vi "ESA-C Move Absolute.vi"(1 "Running":refnum<vi>, 3 "Drive New Abs. Positions":T1={"Drive X Set"=10.0, "Drive Y Set"=10.0, "Drive Z Set"=10.0} {"Drive X Set" min=10.0 max=160.0 step=0.1 format="%.1f"; "Drive Z Set" min=10.0 max=160.0 step=0.1 format="%.1f"; "Drive Y Set" min=10.0 max=160.0 step=0.1 format="%.1f"}, 4 "Drive Connection Settings":T2={"Objective GPIB-Port"=4, "Stage GPIB-Port"=4, "Drive Selector"=0, "Drive Velocity (V/s)"=5.0} {"Drive Velocity (V/s)" min=10.0 max=160.0 step=0.1 format="%.1f"; "Drive Selector" items=["Obj.", "Stage"]; "Stage GPIB-Port" min=1 max=20 step=1 format="%#.0f"; "Objective GPIB-Port" min=1 max=20 step=1 format="%#.0f"}) -> ()   [LabVIEW 2010]
uses:
  TypeDefs/ESA-C Connection Settings.ctl
  TypeDefs/ESA-C Set Positions.ctl
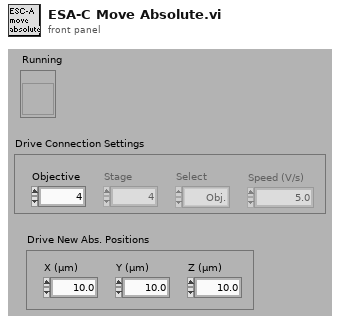
[diagram p1: front panel]
types:
  T1 = typedef "ESA-C Set Positions.ctl" = cluster{"Drive X Set":dbl, "Drive Y Set":dbl, "Drive Z Set":dbl}
  T2 = typedef "ESA-C Connection Settings.ctl" = cluster{"Objective GPIB-Port":i32, "Stage GPIB-Port":i32, "Drive Selector":u16, "Drive Velocity (V/s)":dbl}
  T3 = typedef "ESA-C Current Values.ctl" = cluster{"Voltages":cluster{"Drive X Voltage":dbl, "Drive Y Voltage":dbl, "Drive Z Voltage":dbl}, "Position":cluster{"Drive X Position":dbl, "Drive Y Position":dbl, "Drive Z Position":dbl}}
  T4 = cluster{"Drive X Voltage":dbl, "Drive Y Voltage":dbl, "Drive Z Voltage":dbl}
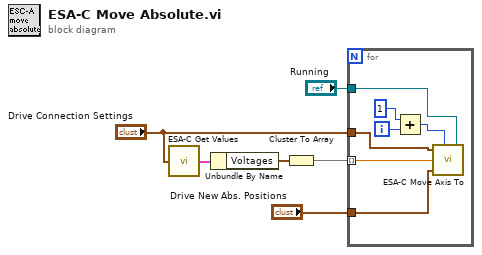
[diagram p0: block diagram]
diagram:
  n1 = call "ESA-C Get Values.vi"("Drive Connection Settings"="Drive Connection Settings") -> ("Drive Current Values"=w6:T3)
  n2 = Unbundle By Name(w6) -> ("Voltages"=w5:T4)
  n3 = Cluster To Array(cluster=w5) -> (array=w4:dbl[])
  n4 = for {
    tunnel: w4 -> [w10] mode=indexing
    tunnel: "Drive New Abs. Positions" -> [w9]
    tunnel: "Drive Connection Settings" -> [w8]
    tunnel: "Running" -> [w7]
    i -> [w12]
    n5 = Add(x=1, y=w12) -> (x+y=w11:i32)
    n6 = call "ESA-C Move Axis To.vi"("Drive Connection Settings"=w8, "Axis"=w11, "Current Voltage (V)"=w10, "Drive New Abs. Positions"=w9, "Running"=w7) -> ()  [unwired: 2 in]
  }
